vi "Send Search Results.vi"(7 "Message Priority (Normal)":T1=enum."Normal", 8 "error in (no error)":errorcluster, 9 "Search Results":string[][](table), 10 "Actor Name":string, 11 "Message Enqueuer":refnum<class "Message Enqueuer.lvclass">) -> (0 "error out":errorcluster, 3 "Message Enqueuer out":refnum<class "Message Enqueuer.lvclass">)   [LabVIEW 2021, in "DB_Search Results.lvlib" / "Search Results Msg.lvclass"]
doc: "This VI sends the message to an actor."
uses:
  <userlib>/John_Lib/Interfaces/DB_Search Results Messages/Search Results Msg/Search Results Msg.lvclass
  <vilib>/ActorFramework/Message Enqueuer/Message Enqueuer.lvclass
  <vilib>/ActorFramework/Message Enqueuer/Message Priority.ctl
  C:/Program Files (x86)/National Instruments/LabVIEW 2021/vi.lib/ActorFramework/Message/Message.lvclass
  <userlib>/John_Lib/Interfaces/DB_Search Results Messages/Search Results Msg/Search Results Msg.lvclass/Search Results Msg.ctl
  <vilib>/ActorFramework/Message Enqueuer/Message Enqueuer.lvclass/Message Enqueuer.ctl
  <vilib>/ActorFramework/Message Priority Queue/Priority Enqueue.vi
  C:/Program Files (x86)/National Instruments/LabVIEW 2021/user.lib/John_Lib/Interfaces/DB_Search Results Messages/Search Results Msg/Search Results Msg.lvclass
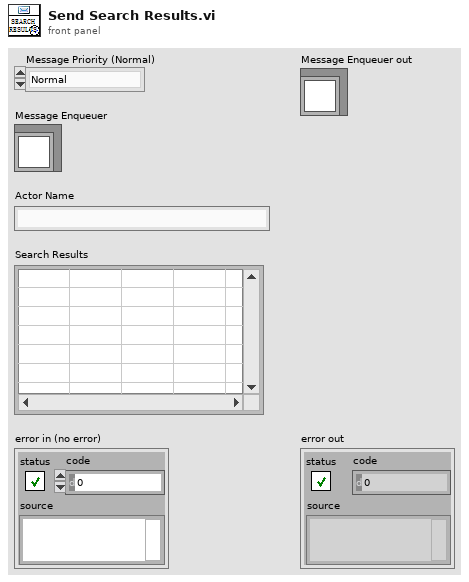
[diagram p1: front panel]
types:
  T1 = typedef "Actor Framework.lvlib/Message Enqueuer.lvclass/Message Priority.ctl" = enum16{"Low", "Normal", "High"}
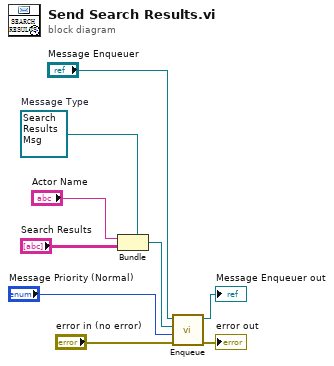
[diagram p0: block diagram]
diagram:
  w6 = refnum<class "Search Results Msg.lvclass"> refnum  # Message Type
  n1 = Bundle(cluster=w6, "Actor Name", "Search Results") -> (w5:refnum<class "Search Results Msg.lvclass">)
  n2 = call <vilib>:"Enqueue.vi"("error in (no error)"="error in (no error)", "Message Priority (Normal)"="Message Priority (Normal)", "Message"=w5, "Message Enqueuer in"="Message Enqueuer") -> ("error out"=→"error out":errorcluster, "Message Enqueuer in"=→"Message Enqueuer out":refnum<class "Message Enqueuer.lvclass">)  [unwired: 6 in]
